vi "Set Sensor.vi"(8 "error in (no error)":errorcluster, 9 "Sensor DAO In":refnum<class "Sensor DAO Class.lvclass">, 10 "Name":string, 11 "Sensor List Class in":refnum<class "Sensor List Class.lvclass">) -> (0 "error out":errorcluster, 3 "Sensor List Class out":refnum<class "Sensor List Class.lvclass">)   [LabVIEW 2013, in "Sensor List Class.lvclass"]
uses:
  Sensor List Class.lvclass
  W:/NSEL OM/lib/Data Access Objects/Sensors/Sensor DAO Class.lvclass
  Sensor List Class.lvclass/Sensor List Class.ctl
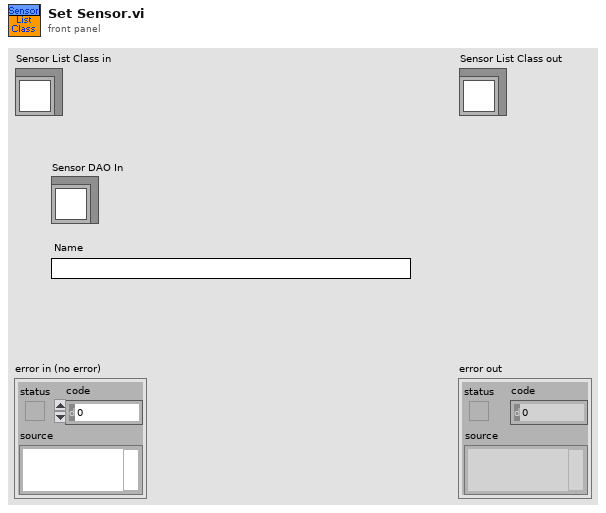
[diagram p1: front panel]
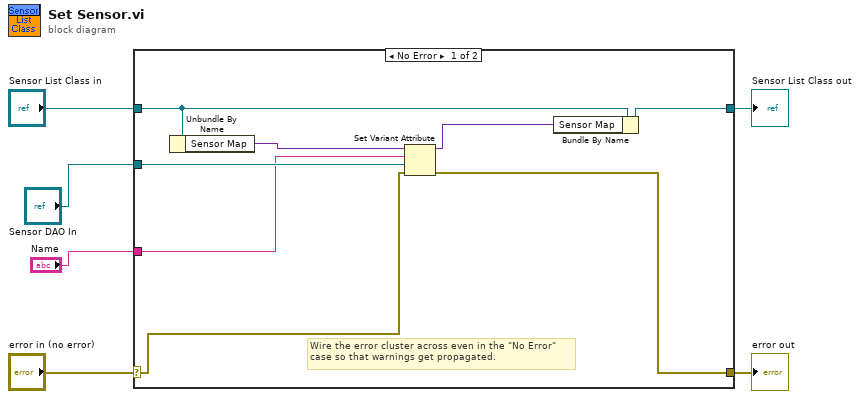
[diagram p0: block diagram]
diagram:
  n1 = case shown="No Error" "error in (no error)" {
    selector: "error in (no error)" -> [w14 w16]
    tunnel: [w13 w16] -> w5
    tunnel: [w8 w15] -> w3
    tunnel: "Sensor List Class in" -> [w12 w15]
    tunnel: "Sensor DAO In" -> [w10 _]
    tunnel: "Name" -> [w9 _]
    frame No Error {
      # "Wire the error cluster across even in the \"No Error\"\ncase so that warnings get propagated."
      n2 = Unbundle By Name(w12) -> ("Sensor Map"=w11:variant)
      n3 = Set Variant Attribute(Variant=w11, name=w9, value=w10, error in=w14) -> (Variant out=w7:variant, error out=w13:errorcluster)  [unwired: 1 out]
      n4 = Bundle By Name(cluster=w12, "Sensor Map"=w7) -> (w8:refnum<class "Sensor List Class.lvclass">)
    }
    frame Error {
    }
  }
  "error out" <- w5
  "Sensor List Class out" <- w3
